vi "Memory.Pointer.Errors.Null Pointer.vi"(7 "source vi name":string, 8 "error in (no error)":errorcluster, 11 "pointer in":refnum<class "Memory.Pointer.lvclass">) -> (0 "error out":errorcluster, 3 "pointer out":refnum<class "Memory.Pointer.lvclass">)   [LabVIEW 2016, in "Memory.lvlib" / "Memory.Pointer.lvclass"]
uses:
  Memory.Pointer.lvclass
  Memory.Pointer.Errors.ctl
  Submodules/SEH/Source/VIs/Static Error Handling.Error Cluster Constant.vi
  Submodules/SEH/Source/VIs/Static Error Handling.Error Cluster Constant (256B).vi
  Submodules/SEH/Source/VIs/Static Error Handling.Parameters.Status.Set.vi
  Submodules/SEH/Source/VIs/Static Error Handling.Parameters.Code.Set.vi
  Submodules/SEH/Source/VIs/Static Error Handling.Parameters.VI Source.Set.vi
  Constants/Memory.Constants.vi
  Constants/Memory.Constants.Library Name.vi
  Memory.Pointer.Errors.Get Info.vi
  Submodules/SEH/Source/VIs/Static Error Handling.Source Buffer.Write.String.vi
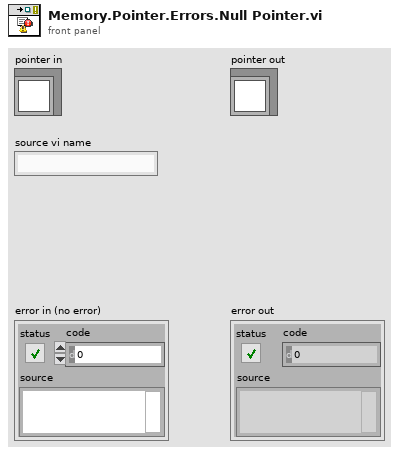
[diagram p1: front panel]
types:
  T1 = typedef "Memory.lvlib/Memory.Pointer.lvclass/Memory.Pointer.Errors.ctl" = enum16{"Out of Bounds", "Buffer Underflow", "Size Mismatch", "Zone", "Null Pointer"}
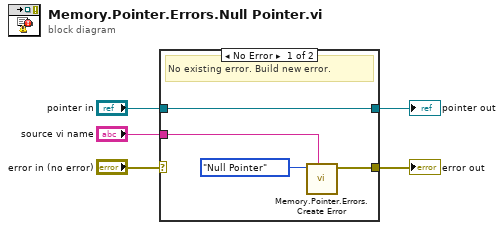
[diagram p0: block diagram]
diagram:
  n1 = case shown="No Error" "error in (no error)" {
    selector: "error in (no error)" -> [_ w11]
    tunnel: [w6 w11] -> w3
    tunnel: "source vi name" -> [w8 _]
    tunnel: "pointer in" -> [w7 w10]
    tunnel: [w7 w10] -> w1
    frame No Error {
      # "No existing error. Build new error."
      n2 = call "Memory.Pointer.Errors.Create Error.vi"("source vi name"=w8, "error"=Memory.Pointer.Errors."Null Pointer") -> ("error out"=w6:errorcluster)  [unwired: 8 in, 1 out]
    }
    frame Error {
      # "Incoming error. Pass through."
    }
  }
  "error out" <- w3
  "pointer out" <- w1
